vi "Start All.vi"(8 "error in":errorcluster, 9 "start configuration (all)":T1={"Start the monitor? (true)"=TRUE, "Start the remote terminals? (true)"=TRUE, "Start the bus controller? (true)"=TRUE}, 10 "bus controller transfer settings (default)":T2={"Start Mode (immediate)"=enum."Immediate", "Count (0 = infinite)"=0, "Minor Frame Time (1 msec)"=0.001, "Start Address (0)"=0} {"Start Address (0)" format="%08x"; "Minor Frame Time (1 msec)" min=0.001 max=1048.576 step=0.001 format="%.3f"}, 11 "module handle":u32) -> (0 "error out":errorcluster, 3 "module handle out":u32)   [LabVIEW 2020, in "AIM MIL-STD-1553 Hardware API.lvlib"]
doc: "<B>Input Parameters:</B>\n\nModule Handle - Reference to the device as obtained from a call to: 1553 General - Obtain a Device Reference.vi\n\nBIU Number (1) - BIU number (one-based) of the bus interface unit.\n\n<B> Output Parameters: </B>"
uses:
  AIM MIL-STD-1553 Hardware API.lvlib
  <instrlib>/_AIM MIL-STD-1553/AIM Controls/1553 BC Transfer Settings.ctl
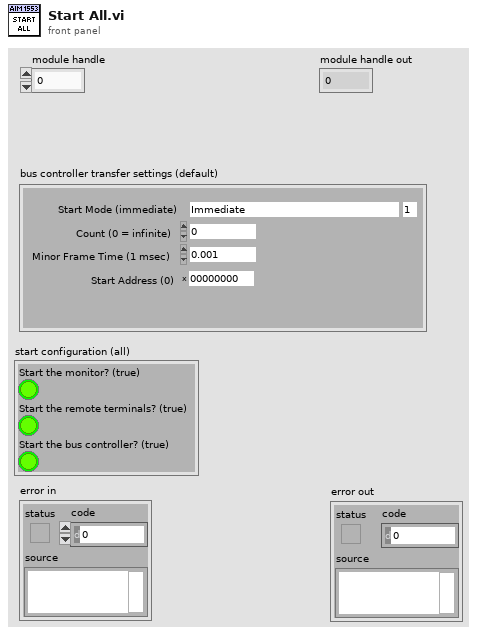
[diagram p1: front panel]
types:
  T1 = cluster{"Start the monitor? (true)":bool, "Start the remote terminals? (true)":bool, "Start the bus controller? (true)":bool}
  T2 = typedef "1553 BC Transfer Settings.ctl" = cluster{"Start Mode (immediate)":enum16{"undefined", "Immediate", "External trigger", "Mode code dynamic bus control", "External pulse", "Setup for fast start", "Fast start", "Start instruction table", "Continue instruction table"}, "Count (0 = infinite)":u32, "Minor Frame Time (1 msec)":sgl, "Start Address (0)":u32}
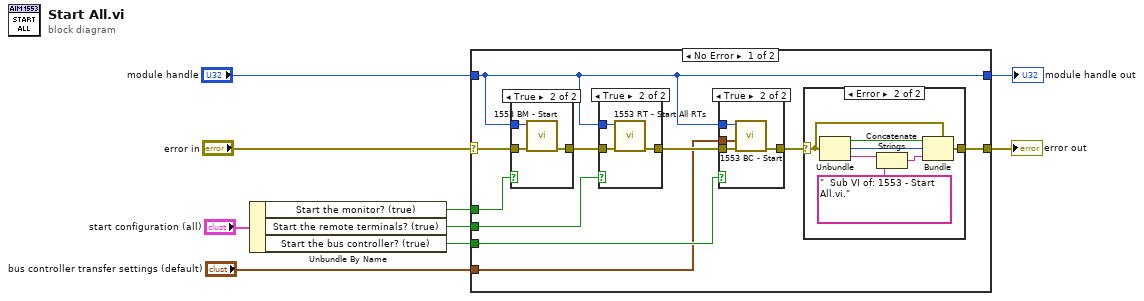
[diagram p0: block diagram]
diagram:
  n1 = Unbundle By Name("start configuration (all)") -> ("Start the monitor? (true)"=w5:bool, "Start the remote terminals? (true)"=w4:bool, "Start the bus controller? (true)"=w3:bool)
  n2 = case shown="No Error" "error in" {
    selector: "error in" -> [w19 w42]
    tunnel: [w15 w42] -> w8
    tunnel: "module handle" -> [w10 w41]
    tunnel: w5 -> [w14 _]
    tunnel: w4 -> [w13 _]
    tunnel: w3 -> [w12 _]
    tunnel: "bus controller transfer settings (default)" -> [w11 _]
    tunnel: [w10 w41] -> w1
    frame No Error {
      n3 = case shown="True" w14 {
        tunnel: w19 -> [w29 w32]
        tunnel: [w29 w31] -> w18
        tunnel: w10 -> [_ w30]
        frame False {
        }
        frame True {
          n4 = call <instrlib>:"1553 BM - Start.vi"("Error In (none)"=w32, "Module Handle"=w30) -> ("Error Out"=w31:errorcluster)  [unwired: 8 in, 1 out]
        }
      }
      n5 = case shown="True" w13 {
        tunnel: w18 -> [w25 w28]
        tunnel: [w25 w27] -> w17
        tunnel: w10 -> [_ w26]
        frame False {
        }
        frame True {
          n6 = call <instrlib>:"1553 RT - Start All RTs.vi"("Error In (none)"=w28, "Module Handle"=w26) -> ("Error Out"=w27:errorcluster)  [unwired: 8 in, 1 out]
        }
      }
      n7 = case shown="True" w12 {
        tunnel: w17 -> [w20 w24]
        tunnel: w10 -> [_ w23]
        tunnel: [w20 w22] -> w16
        tunnel: w11 -> [_ w21]
        frame False {
        }
        frame True {
          n8 = call <instrlib>:"1553 BC - Start.vi"("Error In (none)"=w24, "BC Transfersettings"=w21, "Module Handle"=w23) -> ("Error Out"=w22:errorcluster)  [unwired: 5 in, 3 out]
        }
      }
      n9 = case shown="Error" w16 {
        selector: w16 -> [w33 w40]
        tunnel: [w33 w37] -> w15
        frame No Error {
        }
        frame Error {
          n10 = Unbundle(w40) -> ("status"=w38:bool, "code"=w39:i32, "source"=w36:string)
          n11 = Concatenate Strings(w36, "  Sub VI of: 1553 - Start All.vi.") -> (w35:string)
          n12 = Bundle(cluster=w40, "status"=w38, "code"=w39, "source"=w35) -> (w37:errorcluster)
        }
      }
    }
    frame Error {
    }
  }
  "error out" <- w8
  "module handle out" <- w1
